vi "VI Tree.vi"   [LabVIEW 2013, in "Thorlabs_MC2000B.lvlib"]
uses:
  <instrlib>/Thorlabs_MC2000B/Thorlabs_MC2000B.lvlib
panel:
  # "(c) 2009 <Enter Company Name Here>.  ALL RIGHTS RESERVED."
  # "SEE DIAGRAM\nFOR VI TREE."
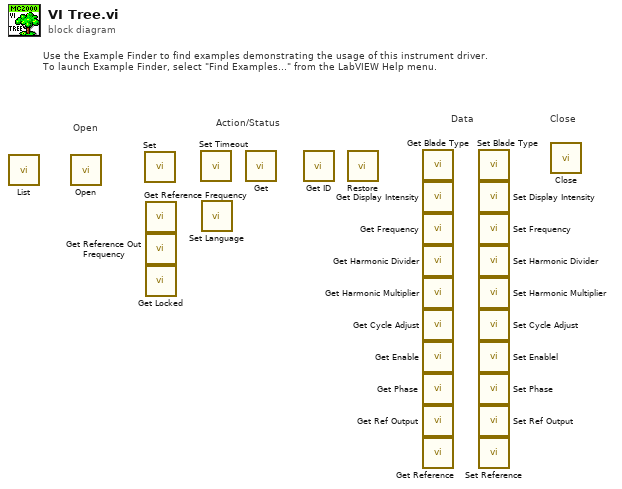
[diagram p0: block diagram]
diagram:
  # "Data"
  # "Action/Status"
  # "Close"
  # "Open"
  # "Use the Example Finder to find examples demonstrating the usage of this instrument driver.\nTo launch Example Finder, select \"Find Examples...\" from the LabVIEW Help menu."
  n1 = call <instrlib>:"List.vi"() -> ()  [unwired: 8 in, 4 out]
  n2 = call <instrlib>:"Open.vi"() -> ()  [unwired: 9 in, 3 out]
  n3 = call <instrlib>:"Set.vi"() -> ()  [unwired: 10 in, 2 out]
  n4 = call <instrlib>:"Get Reference Frequency.vi"() -> ()  [unwired: 9 in, 3 out]
  n5 = call <instrlib>:"Get Reference Out Frequency.vi"() -> ()  [unwired: 9 in, 3 out]
  n6 = call <instrlib>:"Get Locked.vi"() -> ()  [unwired: 9 in, 3 out]
  n7 = call <instrlib>:"Set Timeout.vi"() -> ()  [unwired: 10 in, 2 out]
  n8 = call <instrlib>:"Set Language.vi"() -> ()  [unwired: 10 in, 2 out]
  n9 = call <instrlib>:"Get.vi"() -> ()  [unwired: 9 in, 3 out]
  n10 = call <instrlib>:"Get ID.vi"() -> ()  [unwired: 9 in, 3 out]
  n11 = call <instrlib>:"Restore.vi"() -> ()  [unwired: 11 in, 1 out]
  n12 = call <instrlib>:"Get Blade Type.vi"() -> ()  [unwired: 9 in, 3 out]
  n13 = call <instrlib>:"Get Display Intensity.vi"() -> ()  [unwired: 9 in, 3 out]
  n14 = call <instrlib>:"Get Frequency.vi"() -> ()  [unwired: 9 in, 3 out]
  n15 = call <instrlib>:"Get Harmonic Divider.vi"() -> ()  [unwired: 9 in, 3 out]
  n16 = call <instrlib>:"Get Harmonic Multiplier.vi"() -> ()  [unwired: 9 in, 3 out]
  n17 = call <instrlib>:"Get Cycle Adjust.vi"() -> ()  [unwired: 9 in, 3 out]
  n18 = call <instrlib>:"Get Enable.vi"() -> ()  [unwired: 9 in, 3 out]
  n19 = call <instrlib>:"Get Phase.vi"() -> ()  [unwired: 9 in, 3 out]
  n20 = call <instrlib>:"Get Ref Output.vi"() -> ()  [unwired: 9 in, 3 out]
  n21 = call <instrlib>:"Get Reference.vi"() -> ()  [unwired: 9 in, 3 out]
  n22 = call <instrlib>:"Set Blade Type.vi"() -> ()  [unwired: 10 in, 2 out]
  n23 = call <instrlib>:"Set Display Intensity.vi"() -> ()  [unwired: 10 in, 2 out]
  n24 = call <instrlib>:"Set Frequency.vi"() -> ()  [unwired: 10 in, 2 out]
  n25 = call <instrlib>:"Set Harmonic Divider.vi"() -> ()  [unwired: 10 in, 2 out]
  n26 = call <instrlib>:"Set Harmonic Multiplier.vi"() -> ()  [unwired: 10 in, 2 out]
  n27 = call <instrlib>:"Set Cycle Adjust.vi"() -> ()  [unwired: 10 in, 2 out]
  n28 = call <instrlib>:"Set Enablel.vi"() -> ()  [unwired: 10 in, 2 out]
  n29 = call <instrlib>:"Set Phase.vi"() -> ()  [unwired: 10 in, 2 out]
  n30 = call <instrlib>:"Set Ref Output.vi"() -> ()  [unwired: 10 in, 2 out]
  n31 = call <instrlib>:"Set Reference.vi"() -> ()  [unwired: 10 in, 2 out]
  n32 = call <instrlib>:"Close.vi"() -> ()  [unwired: 11 in, 1 out]
